vi "VISA_Write_Keysight.vi"(7 "VISA CMD":string="SYST:PRES", 8 "error in":errorcluster, 11 "VISA in":refnum<visa-resource-name>) -> (0 "error out":errorcluster, 3 "VISA out":refnum<visa-resource-name>)   [LabVIEW 2023, in "Keysight.lvlib"]
uses:
  Keysight.lvlib
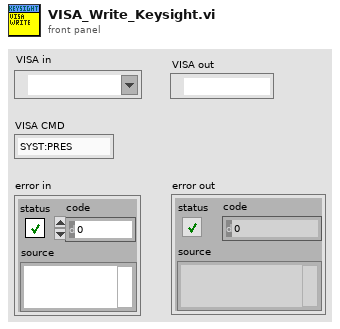
[diagram p1: front panel]
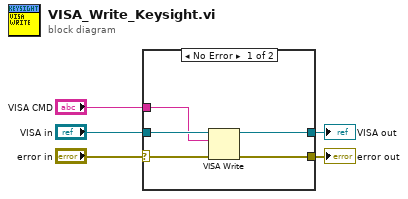
[diagram p0: block diagram]
diagram:
  n1 = case shown="No Error" "error in" {
    selector: "error in" -> [w10 w11]
    tunnel: "VISA in" -> [w9 w12]
    tunnel: "VISA CMD" -> [w8 _]
    tunnel: [w7 w12] -> w2
    tunnel: [w6 w11] -> w1
    frame No Error {
      n2 = VISA Write(VISA resource name=w9, write buffer=w8, error in (no error)=w10) -> (VISA resource name out=w7:refnum<visa-resource-name>, error out=w6:errorcluster)  [unwired: 1 out]
    }
    frame Error {
    }
  }
  "VISA out" <- w2
  "error out" <- w1
